vi "Radius Search Byte.vi"(0 "KD Tree Byte in":refnum<class "KD Tree Byte.lvclass">, 1 "Radius":sgl=1.0, 3 "Max Neighbors":i32=1, 5 "Points":u8[][](array[numeric]), 11 "error in (no error)":errorcluster) -> (4 "KD Tree Byte out":refnum<class "KD Tree Byte.lvclass">, 6 "Indices":i32[][](array[numeric]), 8 "Dists":sgl[][](array[numeric]), 10 "N Found":i32[](array[numeric]), 15 "error out":errorcluster)   [LabVIEW 2020, in "KD Tree.lvlib" / "KD Tree Byte.lvclass"]
uses:
  KD Tree Byte.lvclass
  E:/Labview/LV 2020/Libs/flann/flann/Classes/KD Tree/KD Tree.lvclass
  KD Tree/KD Tree.lvclass/KD Tree.ctl
  KD Tree/Read index_ptr.vi
  KD Tree/Read flann_params.vi
  KD Tree/Read Overwrite Lib Path.vi
  KD Tree Byte.lvclass/KD Tree Byte.ctl
  KD Tree.lvlib
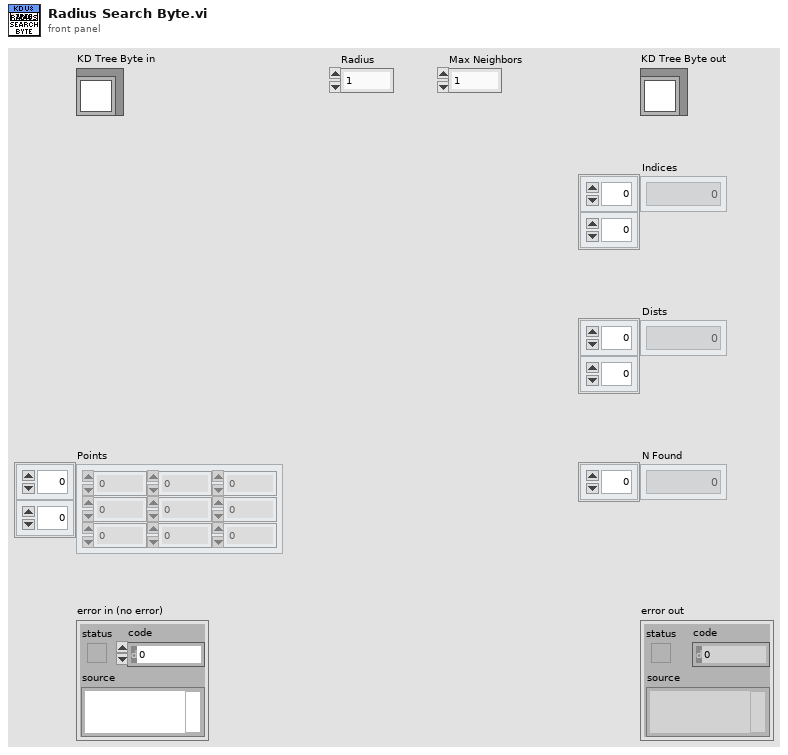
[diagram p1: front panel]
types:
  T1 = typedef "KD Tree.lvlib/Distance Type.ctl" = u32
  T2 = typedef "KD Tree.lvlib/Flann Params.ctl" = cluster{"algorithm":u32, "checks":i32, "eps":sgl, "sorted":i32, "max_neighbors":i32, "cores":i32, "trees":i32, "leaf_max_size":i32, "branching":i32, "iterations":i32, "centers_init":u32, "cb_index":sgl, "target_precision":sgl, "build_weight":sgl, "memory_weight":sgl, "sample_fraction":sgl, "table_number_":u32, "key_size_":u32, "multi_probe_level_":u32, "log_level":u32, "random_seed":i32}
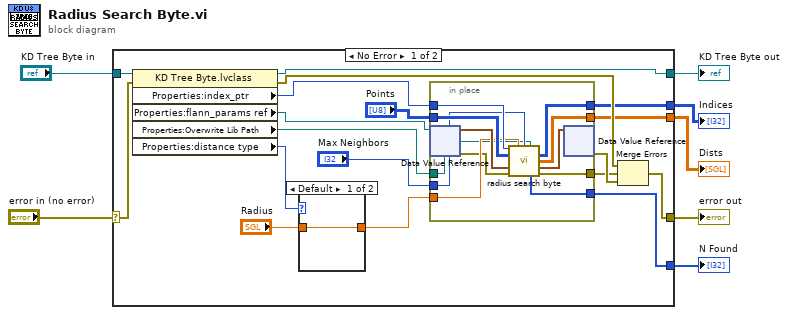
[diagram p0: block diagram]
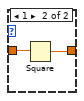
[diagram p2: hidden frame]
diagram:
  n1 = case shown="No Error" "error in (no error)" {
    selector: "error in (no error)" -> [w25 w42]
    tunnel: [w14 w42] -> w4
    tunnel: [w23 w41] -> w5
    tunnel: "KD Tree Byte in" -> [w24 w41]
    tunnel: [w10 _] -> w3
    tunnel: [w9 _] -> w2
    tunnel: [w8 _] -> w1
    frame No Error {
      n2 = property class="KD Tree Byte.lvclass"(reference=w24, error in=w25) -> (reference out=w23:refnum<class "KD Tree Byte.lvclass">, error out=w15:errorcluster, "Properties:index_ptr"=w22:u64, "Properties:flann_params ref"=w21:refnum<data-value>, "Properties:Overwrite Lib Path"=w16:path, "Properties:distance type"=w12:T1)
      n3 = case shown="Default" w12 {
        tunnel: "Radius" -> [w26 w28]
        tunnel: [w26 w27] -> w13
        frame Default {
        }
        frame 1 {
          n4 = Square(x=w28) -> (x^2=w27:sgl)
        }
      }
      n5 = in-place {
        in-place-border: w22 -> [w40]
        in-place-border: "Points" -> [w39]
        in-place-border: [w36] -> w9
        in-place-border: [w35] -> w8
        in-place-border: w13 -> [w34]
        in-place-border: "Max Neighbors" -> [w33]
        in-place-border: [w32] -> w10
        in-place-border: [w31] -> w17
        in-place-border: w16 -> [w29]
        n6 = in-place-dvr #1(w21) -> (w38:T2, w30:errorcluster)
        n7 = call "radius search byte.vi"("index_ptr"=w40, "radius"=w34, "max_nn"=w33, "Overwrite Lib Path"=w29, "query points"=w39, "flann_params"=w38, "error in (no error)"=w30) -> ("indices out"=w35:i32[][], "dists out"=w36:sgl[][], "flann_params"=w37:T2, "N Found"=w32:i32[], "error out"=w31:errorcluster)  [unwired: 3 in, 1 out]
        n8 = in-place-dvr #1(w37) -> (w20:errorcluster)  [unwired: 1 out]
      }
      n9 = Merge Errors(w15, w17, w20) -> (w14:errorcluster)
    }
    frame Error {
    }
  }
  "error out" <- w4
  "KD Tree Byte out" <- w5
  "Indices" <- w1
  "Dists" <- w2
  "N Found" <- w3
